vi "Bin Arrival Time TIO.vi"(0 "Read Position":i32, 1 "Array In":i32[][](array[numeric]), 2 "Thresholding Cluster 2":T1={"F_DEx"=0, "F_AA"=0, " No of Bins"=100}, 3 "Time Bin (s)":dbl=1.0 format="%.2f", 4 "APD Chart 2":refnum<vi>, 5 "Column Definitions":T2(array[cluster]) {"Offset" format="%.2f"; "Resolution" format="%.2f"}, 6 "Histogram In":dbl[][](array[numeric]), 7 "Pulse Width Cluster 2":cluster{dbl, dbl}, 8 "Pulse Widths":cluster{"Pulse Spec 1 (Clocks)":u32, u32}, 9 "Update Time In":dbl format="%.2f", 11 "Binning Position":i32, 12 "Number of Channels":i32, 14 "Intensity Graph":refnum<vi>) -> (10 "Update Time Out":dbl format="%.2f", 13 "Histogram Out":dbl[][](array[numeric]), 15 "Binning Position Out":i32)   [LabVIEW 2009]
panel:
  out "F_DEx":i32
  out "F_AA":i32
  out "Pulse Spec 1 (Clocks)":u32
  out "Numeric 2":dbl
  out "Numeric":dbl
  out "x/y":dbl
  out "nearest integer value":dbl
  out "element 2":dbl
  out "element":dbl
  out "Pulse Width":dbl
  in  "x":dbl=1.0
  out "Array":i32[](array[numeric])
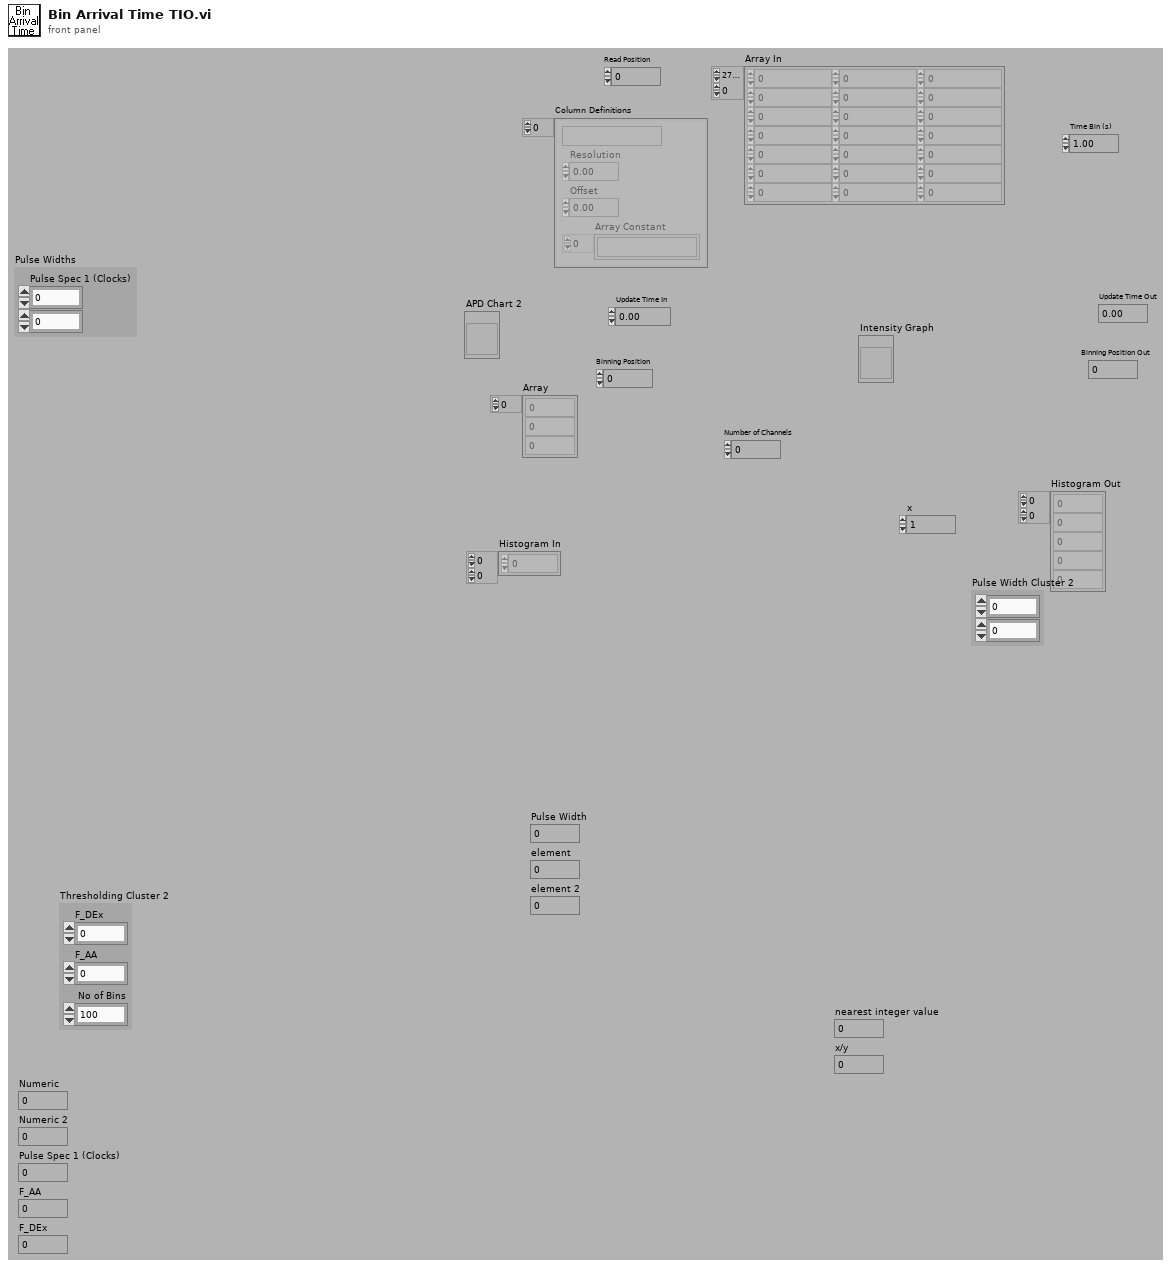
[diagram p1: front panel]
types:
  T1 = cluster{"F_DEx":i32, "F_AA":i32, " No of Bins":i32}
  T2 = cluster{string, "Resolution":dbl, "Offset":dbl, "Array Constant":string[]}[]
  T3 = cluster{string, "Resolution":dbl, "Offset":dbl, "Array Constant":string[]}
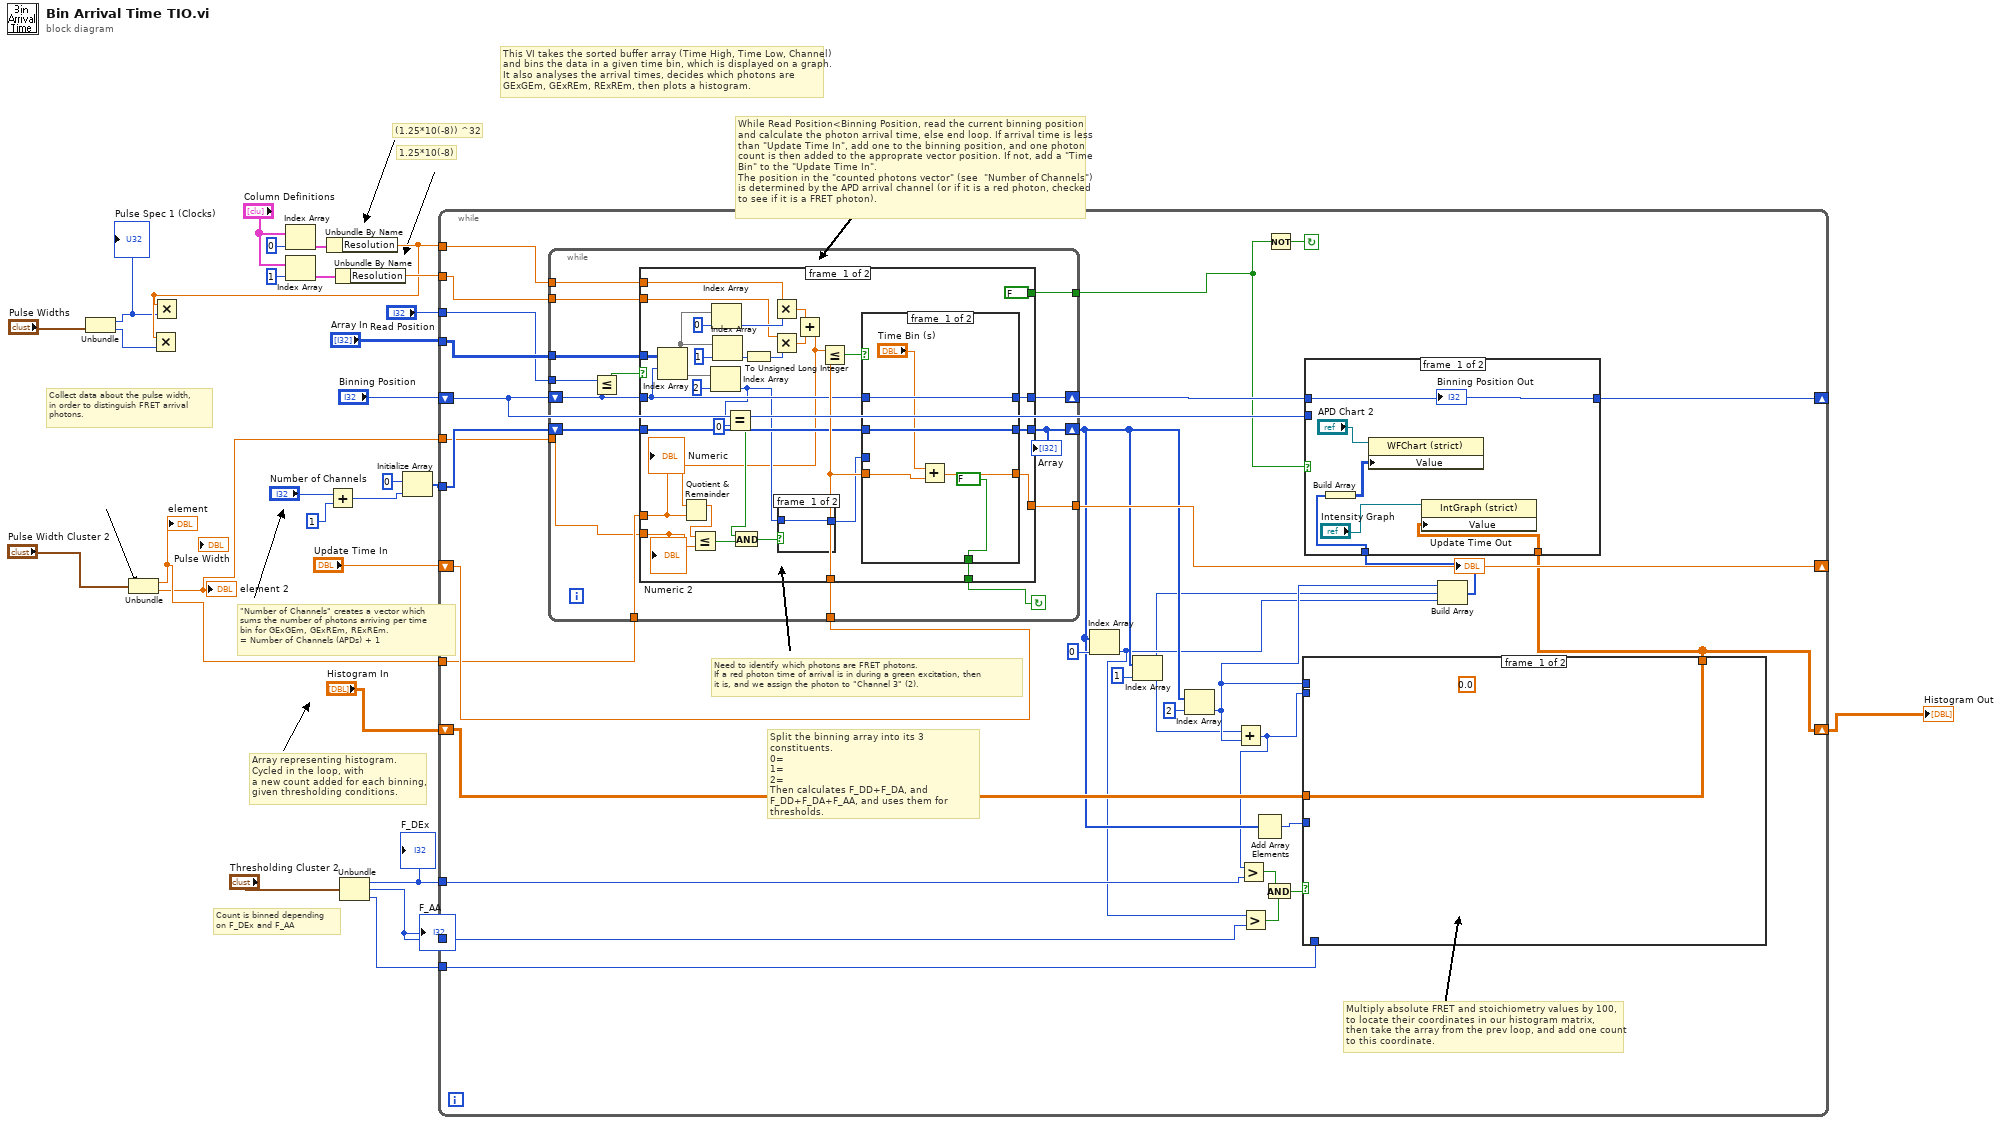
[diagram p0: block diagram]
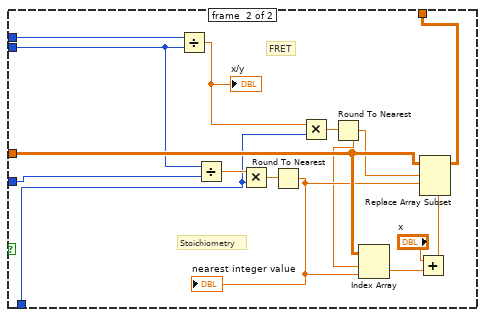
[diagram p2: hidden frame]
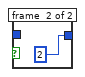
[diagram p3: hidden frame]
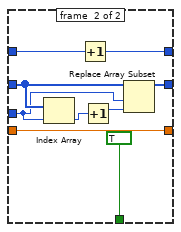
[diagram p4: hidden frame]
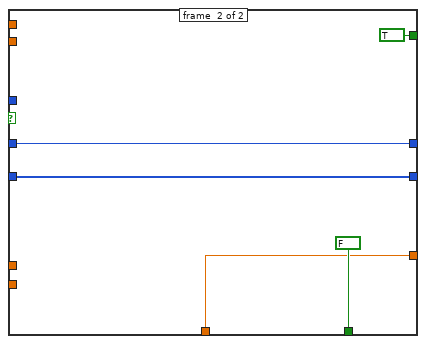
[diagram p5: hidden frame]
diagram:
  # "Count is binned depending\non F_DEx and F_AA"
  # "Collect data about the pulse width,\nin order to distinguish FRET arrival \nphotons."
  # "Array representing histogram.\nCycled in the loop, with\na new count added for each binning, \ngiven thresholding conditions."
  # "\"Number of Channels\" creates a vector which \nsums the number of photons arriving per time \nbin for GExGEm, GExREm, RExREm.\n= Number of Channels (APDs) + 1"
  # "While Read Position<Binning Position, read the current binning position\nand calculate the photon arrival time, else end loop. If arrival time is less \nthan \"Update Time In\", add one to the binning position, and one photon \ncount is then added to the approprate vector position. If not, add a \"Time \nBin\" to the \"Update Time In\". \nThe position in the \"counted photons vector\" (see  \"Number of Channels\")\nis determined by the APD arrival channel (or if it is a red photon, checked\nto see if it is a FRET photon)."
  # "1.25*10(-8)"
  # "(1.25*10(-8)) ^32"
  # "This VI takes the sorted buffer array (Time High, Time Low, Channel)\nand bins the data in a given time bin, which is displayed on a graph.\nIt also analyses the arrival times, decides which photons are\nGExGEm, GExREm, RExREm, then plots a histogram."
  n1 = Unbundle("Pulse Widths") -> ("Pulse Spec 1 (Clocks)"=w6:u32, w5:u32)
  "Pulse Spec 1 (Clocks)" <- w6
  n2 = Unbundle("Pulse Width Cluster 2") -> (w4:dbl, w3:dbl)
  "element" <- w4
  "element 2" <- w3
  n3 = Index Array(array="Column Definitions", index=0 ("Index")) -> (element=w21:T3)
  n4 = Index Array(array="Column Definitions", index=1 ("Index")) -> (element=w19:T3)
  n5 = Unbundle By Name(w21) -> ("Resolution"=w7:dbl)
  n6 = Multiply(x=w7, y=w5) -> ()  [unwired: 1 out]
  n7 = Multiply(x=w7, y=w6) -> ()  [unwired: 1 out]
  n8 = Add(x="Number of Channels", y=1) -> (x+y=w15:i32)
  n9 = Unbundle By Name(w19) -> ("Resolution"=w20:dbl)
  n10 = Unbundle("Thresholding Cluster 2") -> ("F_DEx"=w10:i32, "F_AA"=w9:i32, "No of Bins"=w1:i32)
  "F_AA" <- w9
  "F_DEx" <- w10
  n11 = Initialize Array(0 ("Element Data"), w15) -> (w22:i32[])
  n12 = while {
    tunnel: w22 -> [w54]
    tunnel: w20 -> [w55]
    tunnel: w7 -> [w56]
    tunnel: "Read Position" -> [w57]
    shift-left: "Binning Position" -> [w58]
    shift-right: [w59] -> w29
    shift-left: "Update Time In" -> [w52]
    shift-right: [w51] -> w28
    tunnel: "Array In" -> [w62]
    shift-right: [w47] -> w12
    shift-left: "Histogram In" -> [w46]
    tunnel: w10 -> [w38]
    tunnel: w9 -> [w37]
    tunnel: w4 -> [w36]
    tunnel: w3 -> [w35]
    tunnel: w1 -> [w31]
    stop <- w61 continue-if-true
    # "Multiply absolute FRET and stoichiometry values by 100,\nto locate their coordinates in our histogram matrix,\nthen take the array from the prev loop, and add one count \nto this coordinate."
    # "Split the binning array into its 3 constituents.\n0=\n1=\n2=\nThen calculates F_DD+F_DA, and\nF_DD+F_DA+F_AA, and uses them for \nthresholds."
    # "Need to identify which photons are FRET photons. \nIf a red photon time of arrival is in during a green excitation, then \nit is, and we assign the photon to \"Channel 3\" (2)."
    n13 = while {
      tunnel: [w81] -> w51
      tunnel: w55 -> [w82]
      tunnel: w56 -> [w83]
      tunnel: [w84] -> w53
      tunnel: w57 -> [w88]
      tunnel: w52 -> [w91]
      tunnel: w62 -> [w92]
      shift-left: w54 -> [w90]
      shift-right: [w89] -> w44
      shift-left: w58 -> [w87]
      shift-right: [w93] -> w60
      tunnel: w36 -> [w80]
      tunnel: w35 -> [w79]
      stop <- w85 continue-if-true
      n14 = Less Or Equal?(x=w88, y=w87) -> (x <= y?=w86:bool)
      n15 = case shown="False" w86 {
        tunnel: [w124 w146] -> w93
        tunnel: w92 -> [w116 _]
        tunnel: w87 -> [w117 w146]
        tunnel: w91 -> [w123 w142]
        tunnel: w90 -> [w122 w145]
        tunnel: [w121 w145] -> w89
        tunnel: [w119 FALSE] -> w85
        tunnel: [FALSE TRUE] -> w84
        tunnel: w83 -> [w110 _]
        tunnel: w82 -> [w109 _]
        tunnel: [w106 w142] -> w81
        tunnel: w80 -> [w95 _]
        tunnel: w79 -> [w94 _]
        frame #0 {
          n16 = Index Array(array=w116, index (row)=w117) -> (element=w112:i32[])  [unwired: 1 in]
          n17 = Index Array(array=w112, index=2 ("Index")) -> (element=w102:i32)
          n18 = Index Array(array=w112, index=0 ("Index")) -> (element=w111:i32)
          n19 = Index Array(array=w112, index=1 ("Index")) -> (element=w105:i32)
          n20 = Equal?(x=w102, y=0) -> (x = y?=w99:bool)
          n21 = To Unsigned Long Integer(number=w105) -> (unsigned 32bit integer=w104:u32)
          n22 = Multiply(x=w110, y=w111) -> (x*y=w108:dbl)
          n23 = Multiply(x=w109, y=w104) -> (x*y=w107:dbl)
          n24 = Add(x=w108, y=w107) -> (x+y=w98:dbl)
          n25 = Quotient & Remainder(x=w98, y=w95) -> (x-y*floor(x/y)=w97:dbl)  [unwired: 1 out]
          n26 = Less Or Equal?(x=w97, y=w94) -> (x <= y?=w96:bool)
          n27 = And(x=w99, y=w96) -> (x .and. y?=w100:bool)
          n28 = case shown="False" w100 {
            tunnel: [w125 2 ("Element Data")] -> w103
            tunnel: w102 -> [w125 _]
            frame #0 {
            }
            frame #1 {
            }
          }
          n29 = Less Or Equal?(x=w98, y=w123) -> (x <= y?=w120:bool)
          n30 = case shown="True" w120 {
            tunnel: [w132 w141] -> w124
            tunnel: w117 -> [w132 w140]
            tunnel: [w131 w135] -> w121
            tunnel: w122 -> [w131 w136]
            tunnel: [FALSE TRUE] -> w119
            tunnel: w103 -> [_ w134]
            tunnel: [w129 w133] -> w106
            tunnel: w123 -> [w128 w133]
            frame #0 {
              n31 = Add(x="Time Bin (s)", y=w128) -> (x+y=w129:dbl)
            }
            frame #1 {
              n32 = Index Array(array=w136, index=w134) -> (element=w138:i32)
              n33 = Increment(x=w140) -> (x+1=w141:i32)
              n34 = Increment(x=w138) -> (x+1=w137:i32)
              n35 = Replace Array Subset(array=w136, new element=w137, index=w134) -> (w135:i32[])
            }
          }
          "Numeric" <- w95
          "Numeric 2" <- w94
        }
        frame #1 {
        }
      }
      "Array" <- w89
    }
    n36 = Index Array(array=w44, index=0) -> (element=w33:i32)
    n37 = Index Array(array=w44, index=1) -> (element=w32:i32)
    n38 = Index Array(array=w44, index=2) -> (element=w34:i32)
    n39 = Add(x=w32, y=w34) -> (x+y=w39:i32)
    n40 = Greater?(x=w39, y=w38) -> (0:w42:bool)
    n41 = Greater?(x=w33, y=w37) -> (0:w41:bool)
    n42 = Add Array Elements(numeric array=w44) -> (sum=w43:i32)
    n43 = And(x=w42, y=w41) -> (x .and. y?=w40:bool)
    n44 = Not(x=w53) -> (.not. x?=w61:bool)
    n45 = case shown="True" w40 {
      tunnel: w43 -> [_ w66]
      tunnel: [w63 w76] -> w47
      tunnel: w46 -> [w63 w75]
      tunnel: w39 -> [_ w67]
      tunnel: w34 -> [_ w65]
      tunnel: w31 -> [_ w64]
      frame #0 {
        (unwired) 0.0
      }
      frame #1 {
        # "Stoichiometry"
        # "FRET"
        n46 = Divide(x=w65, y=w67) -> (x/y=w68:dbl)
        "x/y" <- w68
        n47 = Divide(x=w67, y=w66) -> (x/y=w78:dbl)
        n48 = Multiply(x=w78, y=w64) -> (x*y=w77:dbl)
        n49 = Round To Nearest(number=w77) -> (nearest integer value=w74:dbl)
        "nearest integer value" <- w74
        n50 = Multiply(x=w68, y=w64) -> (x*y=w70:dbl)
        n51 = Round To Nearest(number=w70) -> (nearest integer value=w69:dbl)
        n52 = Index Array(array=w75, index (row)=w69, index (col)=w74) -> (element=w72:dbl)
        n53 = Add(x="x", y=w72) -> (x+y=w71:dbl)
        n54 = Replace Array Subset(array=w75, new element=w71, index (row)=w69, index (col)=w74) -> (w76:dbl[][])
      }
    }
    n55 = Build Array(w34, w32, w33) -> (w45:i32[])
    n56 = case shown="False" w53 {
      tunnel: [w152 w153] -> w59
      tunnel: w60 -> [w152 _]
      tunnel: w58 -> [_ w153]
      tunnel: w47 -> [w150 _]
      tunnel: w45 -> [w148 _]
      frame #0 {
        n57 = Build Array(w148) -> (w147:i32[][])
        n58 = property class="WFChart (strict)"(reference="APD Chart 2", "Value"=w147) -> ()  [unwired: 1 in, 2 out]
        n59 = property class="IntGraph (strict)"(reference="Intensity Graph", "Value"=w150) -> ()  [unwired: 1 in, 2 out]
      }
      frame #1 {
      }
    }
  }
  "Binning Position Out" <- w29
  "Update Time Out" <- w28
  "Histogram Out" <- w12
